vi "HDI Bond Pad TL Match.vi"(9 "error in (no error)":errorcluster, 10 "Image Src":T1) -> (0 "error out":errorcluster, 1 "In Range?":bool, 2 "y rel move":dbl, 3 "x rel move":dbl, 4 "Vertical vector":dbl[](array[numeric]), 5 "Angle Between Lines":dbl)   [LabVIEW 2011]
uses:
  <vilib>/vision/Image Controls.llb/IMAQ Image.ctl
  <vilib>/vision/NI_Vision_Development_Module.lvlib
panel:
  in  "Scale Factor":sgl=0.000429
  out "y":sgl
  out "x":sgl
  out "X Coordinate Pixels":dbl
  out "Y Coordinate Pixels":sgl
  out "Remaining Outputs":T2 {"Vertical calibrated"."Point2"."Y" format="%.2f"; "Vertical calibrated"."Point2"."X" format="%.2f"; "Vertical calibrated"."Point1"."Y" format="%.2f"; "Vertical calibrated"."Point1"."X" format="%.2f"; "veritcal"."Point2"."Y" format="%.2f"; "veritcal"."Point2"."X" format="%.2f"; "veritcal"."Point1"."Y" format="%.2f"; "veritcal"."Point1"."X" format="%.2f"; "Edge Coordinates (calibrated) (Straight Edge (Rake) 2)"."Y" format="%.2f"; "Edge Coordinates (calibrated) (Straight Edge (Rake) 2)"."X" format="%.2f"; "Edge Coordinates (Straight Edge (Rake) 2)"."Y" format="%.2f"; "Edge Coordinates (Straight Edge (Rake) 2)"."X" format="%.2f"}
  out "Image Out":T1(plugin-control)
  out "Horizontal Calibrated":T3 {"Point2"."Y" format="%.2f"; "Point2"."X" format="%.2f"; "Point1"."Y" format="%.2f"; "Point1"."X" format="%.2f"}
  out "Hori":cluster{"X":sgl, "Y":sgl}[](array[cluster]) {"Y" format="%.2f"; "X" format="%.2f"}
  out "horizontal rake":T3 {"Point2"."Y" format="%.2f"; "Point2"."X" format="%.2f"; "Point1"."Y" format="%.2f"; "Point1"."X" format="%.2f"}
  out "Edge Coordinates (Straight Edge (Rake) 1)":cluster{"X":sgl, "Y":sgl}[](array[cluster]) {"Y" format="%.2f"; "X" format="%.2f"}
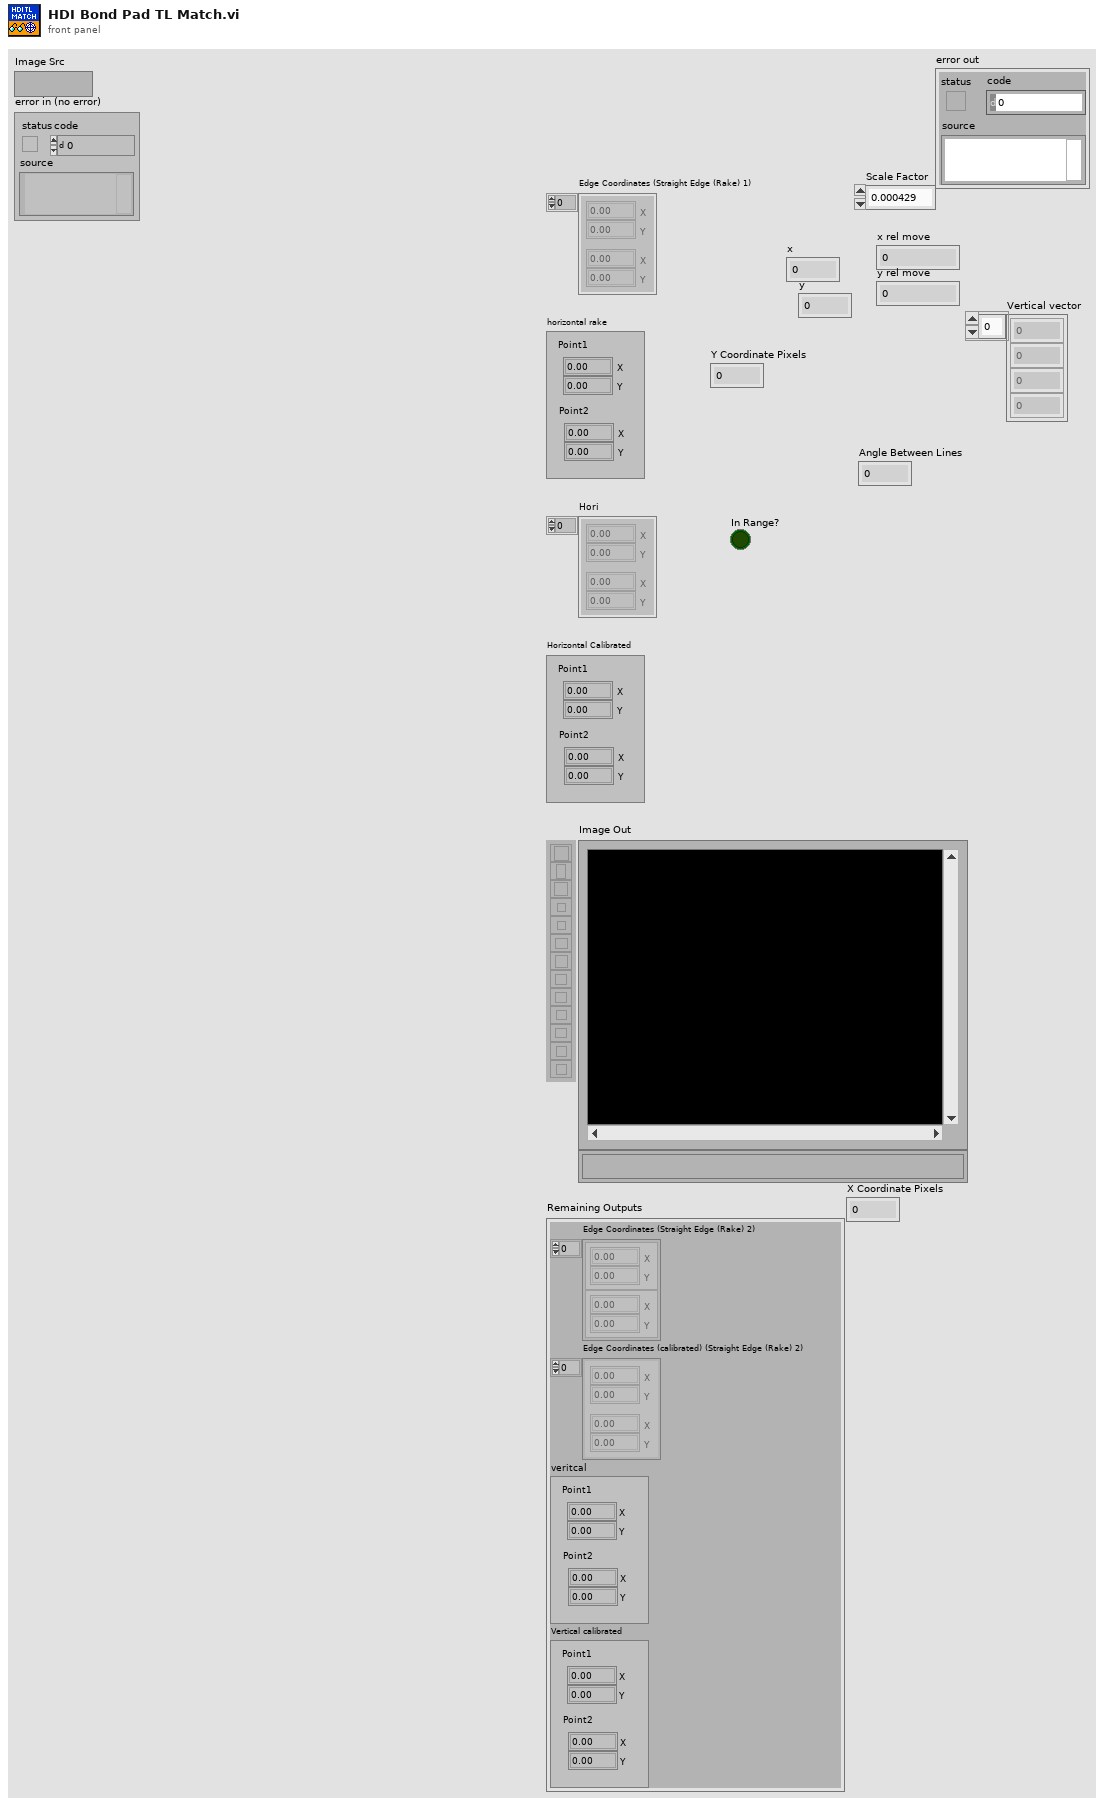
[diagram p1: front panel]
types:
  T1 = typedef "IMAQ Image.ctl" = refnum<image>
  T2 = cluster{"Edge Coordinates (Straight Edge (Rake) 2)":cluster{"X":sgl, "Y":sgl}[], "Edge Coordinates (calibrated) (Straight Edge (Rake) 2)":cluster{"X":sgl, "Y":sgl}[], "veritcal":cluster{"Point1":cluster{"X":sgl, "Y":sgl}, "Point2":cluster{"X":sgl, "Y":sgl}}, "Vertical calibrated":cluster{"Point1":cluster{"X":sgl, "Y":sgl}, "Point2":cluster{"X":sgl, "Y":sgl}}}
  T3 = cluster{"Point1":cluster{"X":sgl, "Y":sgl}, "Point2":cluster{"X":sgl, "Y":sgl}}
  T4 = cluster{"Global Rectangle":i32[], "Contours":cluster{"ID":enum32{"External", "Internal"}, "Type":u32, "Coordinates":i32[]}[]}
  T5 = cluster{"Contrast":i32, "Filter width":i32, "Steepness":i32, "Subsampling Ratio":u32, "Scan Direction":u32, "Show Search Area":bool, "Show Search Lines":bool, "Show Edges Found":bool, "Show Result":bool}
  T6 = typedef "IMAQ Rectangle" = cluster{"Left":i32, "Top":i32, "Right":i32, "Bottom":i32, "Rotation":dbl}
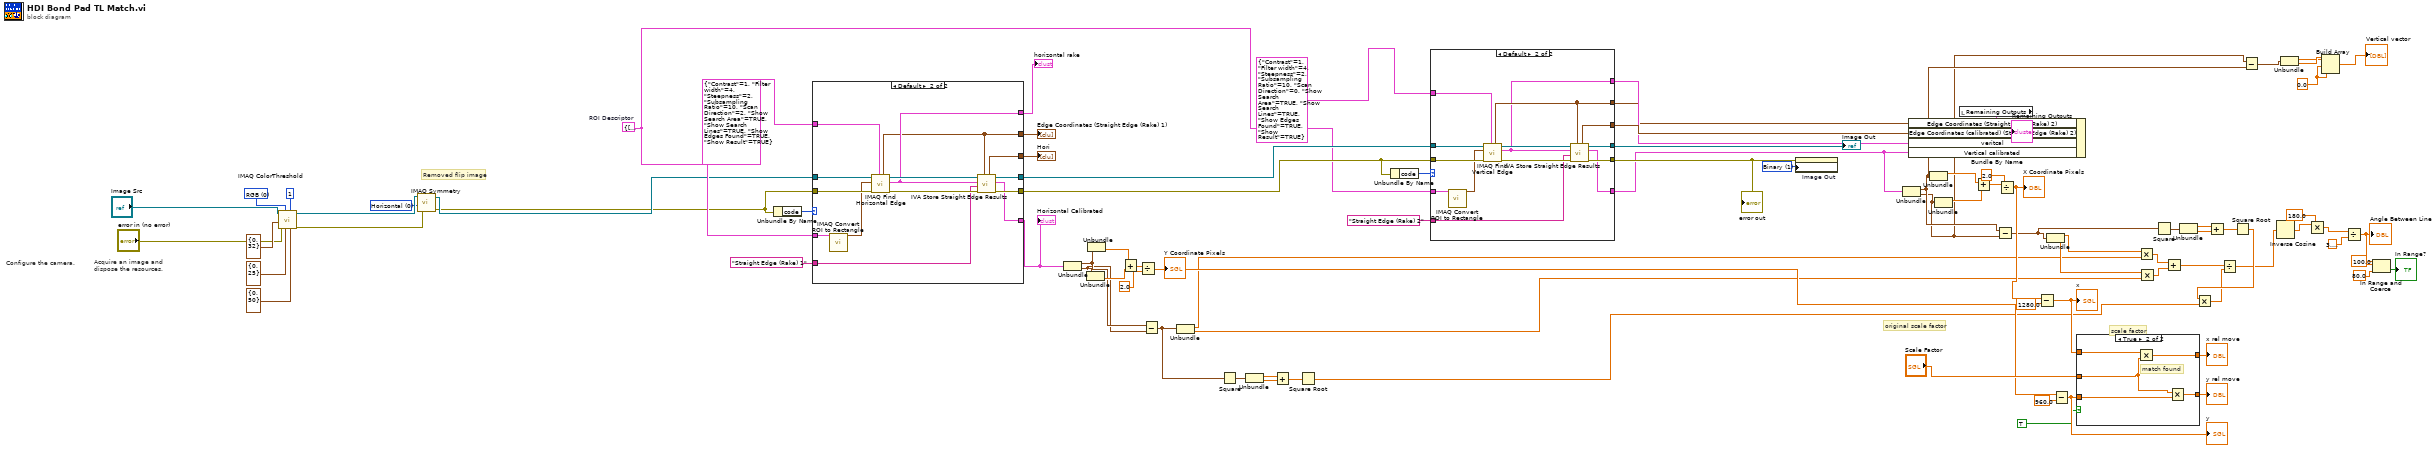
[diagram p0: block diagram]
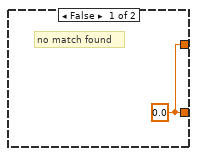
[diagram p2: hidden frame]
diagram:
  w1 = u32 0 items=["Horizontal", "Vertical", "Central", "1st Diagonal", "2nd Diagonal"] ("Type of Symmetry")
  w6 = T4 {"Global Rectangle"=[0, 0, 2650, 1920], "Contours"=[{"ID"=enum."External", "Type"=3, "Coordinates"=[0, 0, 2650, 1920, 0]}]}  # ROI Descriptor
  w14 = 0.0
  w70 = u32 1 items=["Grayscale", "Binary", "Gradient", "Rainbow", "Temperature", "User Defined"] ("Palette")
  w89 = u16 0 items=["RGB", "HSL", "HSV", "HSI"] ("Color Mode")
  # "Removed flip image"
  # "original scale factor"
  # "scale factor"
  # "Acquire an image and\ndispose the resources."
  # "Configure the camera."
  n1 = call "IMAQ ColorThreshold"("Blue or Luma or Val or Inten Range"=cluster{"Lower value":i32, "Upper value":i32} {"Lower value"=0, "Upper value"=50}, "Replace Value"=1, "Green or Sat Range"=cluster{"Lower value":i32, "Upper value":i32} {"Lower value"=0, "Upper value"=25}, "Color Mode"=w89, "error in (no error)"="error in (no error)", "Red or Hue Range"=cluster{"Lower value":i32, "Upper value":i32} {"Lower value"=0, "Upper value"=32}, "Image Src"="Image Src") -> ("error out"=w3:errorcluster, "Image Dst Out"=w5:T1)  [unwired: 3 in]
  n2 = call "IMAQ Symmetry"("error in (no error)"=w3, "Type of Symmetry"=w1, "Image Src"=w5) -> ("error out"=w2:errorcluster, "Image Dst Out"=w4:T1)  [unwired: 2 in]
  n3 = Unbundle By Name(w2) -> ("code"=w79:i32)
  n4 = case shown="Default" w79 {
    tunnel: T5 {"Contrast"=1, "Filter width"=4, "Steepness"=2, "Subsampling Ratio"=10, "Scan Direction"=2, "Show Search Area"=TRUE, "Show Search Lines"=TRUE, "Show Edges Found"=TRUE, "Show Result"=TRUE} ("Settings (Straight Edge (Rake) 1)") -> [_ w105]
    tunnel: w4 -> [w91 w104]
    tunnel: w2 -> [_ w103]
    tunnel: w6 -> [_ w102]
    tunnel: [w91 w99] -> w78
    tunnel: [_ w97] -> w84
    tunnel: [_ w96] -> w83
    tunnel: [_ w95] -> w82
    tunnel: "Straight Edge (Rake) 1" ("Step Name") -> [_ w94]
    tunnel: [_ w93] -> w80
    tunnel: [_ w92] -> w67
    frame -1074396199, -1074396198 {
      # "Discard Coordinate System Error"
    }
    frame Default {
      n5 = call "IMAQ Convert ROI to Rectangle"("ROI Descriptor"=w102) -> ("Rectangle"=w101:T6)  [unwired: 8 in, 1 out]
      n6 = call "IMAQ Find Horizontal Edge"("Settings"=w105, "error in (no error)"=w103, "Rectangle"=w101, "Image"=w104) -> ("error out"=w98:errorcluster, "Line Coordinates"=w96:T3, "Image Out"=w100:T1, "Edge Coordinates"=w95:cluster{"X":sgl, "Y":sgl}[])  [unwired: 2 in, 2 out]
      n7 = call <vilib>:"IVA Store Straight Edge Results.vi"("Edge Coordinates"=w95, "error in (no error)"=w98, "Step Name"=w94, "Line Coordinates"=w96, "Image in"=w100) -> ("error out"=w97:errorcluster, "Line Coordinates (calibrated)"=w92:T3, "Image dup"=w99:T1, "Edge Coordinates (calibrated)"=w93:cluster{"X":sgl, "Y":sgl}[])  [unwired: 3 in]
    }
  }
  "Edge Coordinates (Straight Edge (Rake) 1)" <- w82
  "horizontal rake" <- w83
  "Hori" <- w80
  "Horizontal Calibrated" <- w67
  n8 = Unbundle(w67) -> ("Point1"=w47:cluster{"X":sgl, "Y":sgl}, "Point2"=w46:cluster{"X":sgl, "Y":sgl})
  n9 = Unbundle(w46) -> ("Y"=w65:sgl)  [unwired: 1 out]
  n10 = Unbundle(w47) -> ("Y"=w66:sgl)  [unwired: 1 out]
  n11 = Add(x=w66, y=w65) -> (x+y=w64:sgl)
  n12 = Divide(x=w64, y=sgl 2.0) -> (x/y=w50:sgl)
  "Y Coordinate Pixels" <- w50
  n13 = Subtract(x=w47, y=w46) -> (x-y=w30:cluster{"X":sgl, "Y":sgl})
  n14 = Unbundle(w30) -> ("X"=w43:sgl, "Y"=w42:sgl)
  n15 = Square(x=w30) -> (x^2=w34:cluster{"X":sgl, "Y":sgl})
  n16 = Unbundle(w34) -> ("X"=w33:sgl, "Y"=w32:sgl)
  n17 = Add(x=w33, y=w32) -> (x+y=w31:sgl)
  n18 = Square Root(x=w31) -> (sqrt(x)=w27:sgl)
  n19 = Unbundle By Name(w84) -> ("code"=w72:i32)
  n20 = case shown="Default" w72 {
    tunnel: w78 -> [w106 w120]
    tunnel: w84 -> [_ w119]
    tunnel: T5 {"Contrast"=1, "Filter width"=4, "Steepness"=2, "Subsampling Ratio"=10, "Scan Direction"=0, "Show Search Area"=TRUE, "Show Search Lines"=TRUE, "Show Edges Found"=TRUE, "Show Result"=TRUE} ("Settings (Straight Edge (Rake) 2)") -> [_ w118]
    tunnel: w6 -> [_ w117]
    tunnel: [w106 w114] -> w71
    tunnel: [_ w112] -> w76
    tunnel: [_ w111] -> w9
    tunnel: [_ w110] -> w75
    tunnel: [_ w109] -> w62
    tunnel: [_ w108] -> w74
    tunnel: "Straight Edge (Rake) 2" ("Step Name") -> [_ w107]
    frame -1074396199, -1074396198 {
      # "Discard Coordinate System Error"
    }
    frame Default {
      n21 = call "IMAQ Convert ROI to Rectangle"("ROI Descriptor"=w117) -> ("Rectangle"=w116:T6)  [unwired: 8 in, 1 out]
      n22 = call "IMAQ Find Vertical Edge"("Settings"=w118, "error in (no error)"=w119, "Rectangle"=w116, "Image"=w120) -> ("error out"=w113:errorcluster, "Line Coordinates"=w108:T3, "Image Out"=w115:T1, "Edge Coordinates"=w111:cluster{"X":sgl, "Y":sgl}[])  [unwired: 2 in, 2 out]
      n23 = call <vilib>:"IVA Store Straight Edge Results.vi"("Edge Coordinates"=w111, "error in (no error)"=w113, "Step Name"=w107, "Line Coordinates"=w108, "Image in"=w115) -> ("error out"=w112:errorcluster, "Line Coordinates (calibrated)"=w109:T3, "Image dup"=w114:T1, "Edge Coordinates (calibrated)"=w110:cluster{"X":sgl, "Y":sgl}[])  [unwired: 3 in]
    }
  }
  "Image Out" <- w71
  "error out" <- w76
  n24 = property on="Image Out" class="ImageControl"(error in=w76, "Palette:Palette Type"=w70) -> ()  [unwired: 1 in, 2 out]
  n25 = Unbundle(w62) -> ("Point1"=w8:cluster{"X":sgl, "Y":sgl}, "Point2"=w7:cluster{"X":sgl, "Y":sgl})
  n26 = Unbundle(w8) -> ("X"=w59:sgl)  [unwired: 1 out]
  n27 = Unbundle(w7) -> ("X"=w58:sgl)  [unwired: 1 out]
  n28 = local read "Remaining Outputs"() -> (w68:T2)
  n29 = Bundle By Name(cluster=w68, "Edge Coordinates (Straight Edge (Rake) 2)"=w9, "Edge Coordinates (calibrated) (Straight Edge (Rake) 2)"=w75, "veritcal"=w74, "Vertical calibrated"=w62) -> (→"Remaining Outputs":T2)
  n30 = Add(x=w59, y=w58) -> (x+y=w61:sgl)
  n31 = Subtract(x=w8, y=w7) -> (x-y=w39:cluster{"X":sgl, "Y":sgl})
  n32 = Divide(x=w61, y=2.0) -> (x/y=w49:dbl)
  "X Coordinate Pixels" <- w49
  n33 = Subtract(x=w49, y=sgl 1280.0) -> (x-y=w54:dbl)
  "x" <- w54
  n34 = Unbundle(w39) -> ("X"=w45:sgl, "Y"=w44:sgl)
  n35 = Subtract(x=w50, y=sgl 960.0) -> (x-y=w55:sgl)
  "y" <- w55
  n36 = case shown="True" TRUE {
    tunnel: w55 -> [_ w126]
    tunnel: w54 -> [_ w125]
    tunnel: [w121 w124] -> w53
    tunnel: [w121 w123] -> w52
    tunnel: "Scale Factor" -> [_ w122]
    frame False {
      w121 = sgl 0.0
      # "no match found"
    }
    frame True {
      # "match found"
      n37 = Multiply(x=w125, y=w122) -> (x*y=w124:dbl)
      n38 = Multiply(x=w122, y=w126) -> (x*y=w123:sgl)
    }
  }
  "x rel move" <- w53
  "y rel move" <- w52
  n39 = Multiply(x=w45, y=w43) -> (x*y=w41:sgl)
  n40 = Multiply(x=w44, y=w42) -> (x*y=w40:sgl)
  n41 = Square(x=w39) -> (x^2=w38:cluster{"X":sgl, "Y":sgl})
  n42 = Add(x=w41, y=w40) -> (x+y=w29:sgl)
  n43 = Unbundle(w38) -> ("X"=w37:sgl, "Y"=w36:sgl)
  n44 = Add(x=w37, y=w36) -> (x+y=w35:sgl)
  n45 = Square Root(x=w35) -> (sqrt(x)=w28:sgl)
  n46 = Multiply(x=w28, y=w27) -> (x*y=w26:sgl)
  n47 = Divide(x=w29, y=w26) -> (x/y=w25:sgl)
  n48 = Subtract(x=w7, y=w8) -> (x-y=w12:cluster{"X":sgl, "Y":sgl})
  n49 = Inverse Cosine(1:w25) -> (0:w24:sgl)
  n50 = Unbundle(w12) -> ("X"=w10:sgl, "Y"=w11:sgl)
  n51 = Multiply(x=w24, y=sgl 180.0) -> (x*y=w22:sgl)
  n52 = Build Array(w11, w10, w14, w14) -> (→"Vertical vector":dbl[])
  n53 = Divide(x=w22, y=3.141592653589793) -> (x/y=w20:dbl)
  "Angle Between Lines" <- w20
  n54 = In Range and Coerce(upper limit=100.0, x=w20, lower limit=80.0) -> (In Range?=→"In Range?":bool)  [unwired: 1 out]
